vi "boont_main.vi"(5 "Data File":path, 7 "Command File":path, 8 "error in (no error)":errorcluster, 11 "VISA In":refnum<visa-resource-name>) -> (0 "error out":errorcluster, 2 "Command Num.":dbl, 3 "VISA Out":refnum<visa-resource-name>)   [LabVIEW 2011]
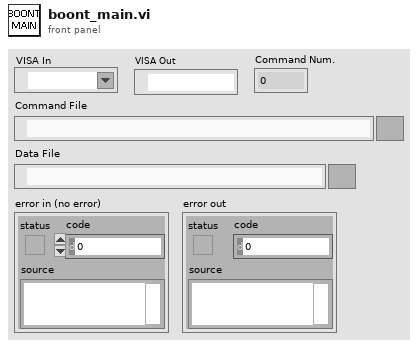
[diagram p1: front panel]
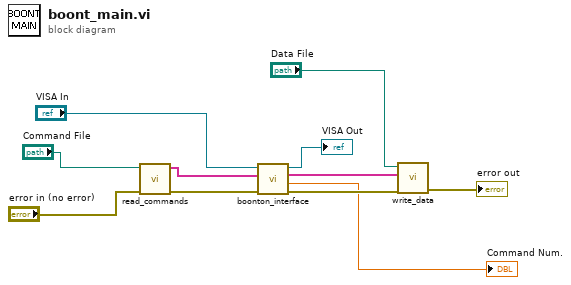
[diagram p0: block diagram]
diagram:
  n1 = call "read_commands.vi"("error in (no error)"="error in (no error)", "Path"="Command File") -> ("error out"=w7:errorcluster, "Command Array"=w5:string[])  [unwired: 8 in]
  n2 = call "boonton_interface.vi"("error in (no error)"=w7, "Command Array"=w5, "VISA In"="VISA In") -> ("error out"=w6:errorcluster, "Command Num."=→"Command Num.":dbl, "Results"=w4:string[], "VISA Out"=→"VISA Out":refnum<visa-resource-name>)  [unwired: 3 in]
  n3 = call "write_data.vi"("error in (no error)"=w6, "Array"=w4, "Data File"="Data File") -> ("error out"=→"error out":errorcluster)  [unwired: 8 in]
